vi "settings.vi"(8 "error in (no error)":errorcluster, 9 "low_resolution?":bool, 11 "reference in":refnum<class "Project Panels.lvclass">) -> (0 "error out":errorcluster, 3 "reference out":refnum<class "Project Panels.lvclass">)   [LabVIEW 2015, in "Project Panels.lvclass"]
uses:
  Project Panels.lvclass
  GUI Controller_llb/state.ctl
  GUI Controller_llb/GUI Controller.lvclass
  SYS/File Controller_llb/File Controller.lvclass
panel:
  out "Title":string
  in  "Number:":string
  in  "Service folder path:":path
  in  "TSR folder path:":path
  in  "not_tracking":bool caption="Notification"
  in  "not_items":bool caption="Notification"
  in  "Tab Control":T1(tab)
  in  "K5:":path
  in  "BB-PFT":path
  in  "RMR-ICU:":path
  in  "Pea Pod:":path
  in  "Bod Pod:":path
  in  "RMR:":path
  in  "CPET:":path
  in  "Fitmate:":path
  in  "K4b2:":path
  in  "K5:2":path caption="K5:"
  in  "BB-PFT 2":path caption="Body Box - PFT:"
  in  "RMR-ICU 2":path caption="RMR-ICU:"
  in  "Pea Pod: 2":path caption="Pea Pod:"
  in  "Bod Pod: 2":path caption="Bod Pod:"
  in  "RMR: 2":path caption="RMR:"
  in  "CPET: 2":path caption="CPET:"
  in  "Fitmate: 2":path caption="Fitmate:"
  in  "K4b2: 2":path caption="K4b2:"
  in  "PartsTracking:":path
  in  "Storage:":path
  in  "Products:":path
  out "StatusBar":string
  in  "Save Button":bool
  in  "Stop Button":bool
  # "Excel Files paths:"
  # "TSR settings:"
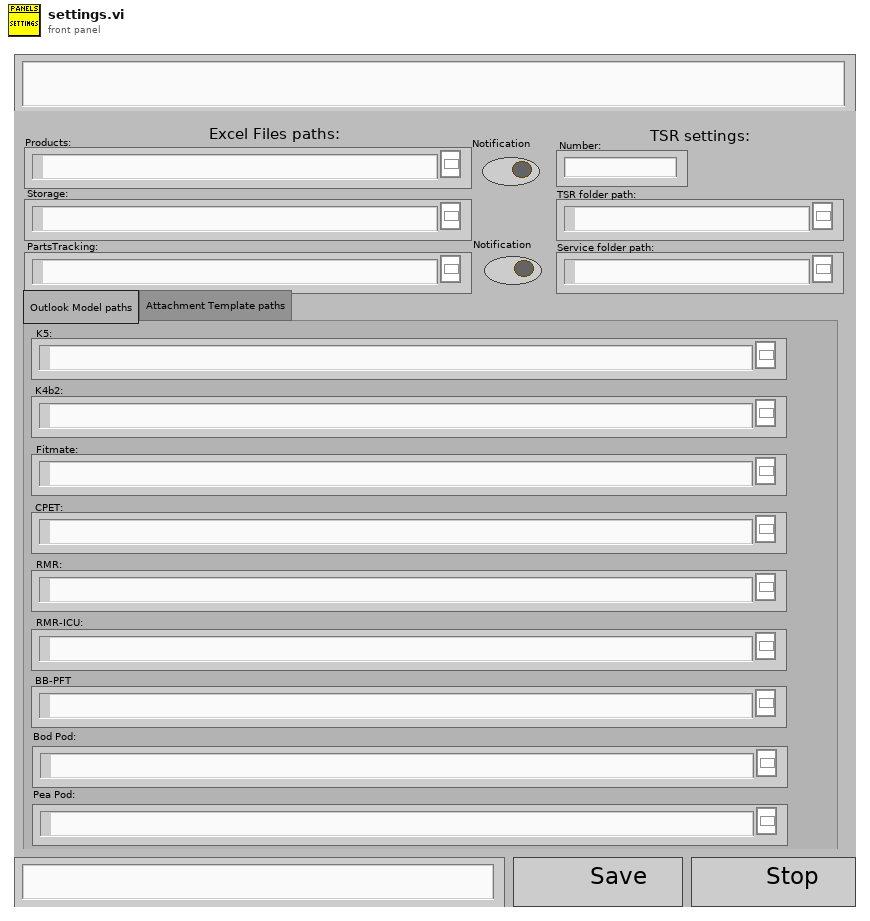
[diagram p1: front panel]
types:
  T1 = enum32{"Outlook Model paths", "Attachment Template paths"}
  T2 = typedef "GUI Controller.lvclass/state.ctl" = enum16{"initiate", "checkNotificationItems", "checkNotificationTracking", "operate", "updateFromFile", "stop"}
  T3 = enum16{"Always On", "Always Off", "Off While Running"}
  T4 = cluster{"number":string, "TSR_path":path, "service_path":path}
  T5 = typedef "Project Panels.lvclass/ObjectAttributesRef.ctl" = refnum<data-value>
  T6 = typedef "Project Panels.lvclass/ObjectAttributes.ctl" = cluster{"MyAttribute":dbl, "device_controller_ref":refnum<class "Devices Controller.lvclass">, "file_controller_ref":refnum<class "File Controller.lvclass">, "item_controller_ref":refnum<class "Items Controller.lvclass">, "item_tables":cluster{"checkIN":string[][], "checkOUT":string[][], "storage":string[][]}, "quickbook_table":cluster{"notes":string[][]}, "notification_controller_ref":refnum<class "Notification Controller.lvclass">, "partstracking_controller_ref":refnum<class "PartsTracking Controller.lvclass">, "product_tables":cluster{"k4b2":string[][], "fitmate":string[][], "RMR":string[][], "CPET":string[][], "BP":string[][], "PP":string[][], "k5":string[][], "bb-pft":string[][]}, "rowsColour":u32[], "low_resolution?":bool}
  T7 = cluster{"filePaths":path[], "outlookTemplatePaths":path[], "attachmentTemplatePaths":path[]}
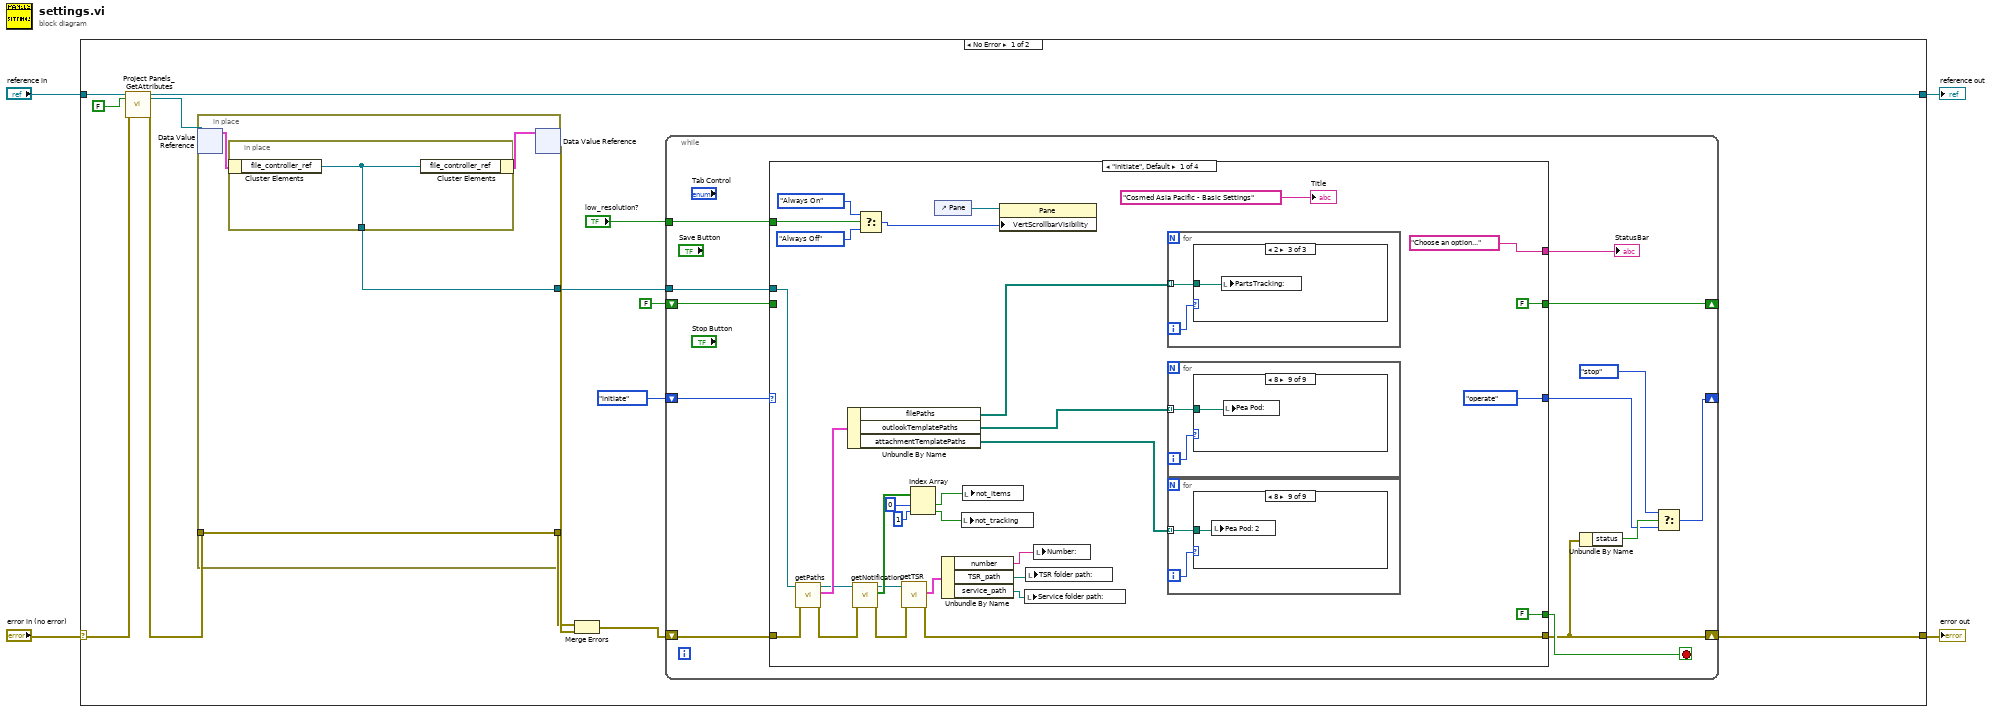
[diagram p0: block diagram]
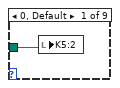
[diagram p2: hidden frame]
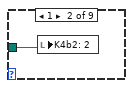
[diagram p3: hidden frame]
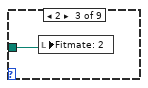
[diagram p4: hidden frame]
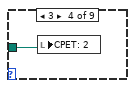
[diagram p5: hidden frame]
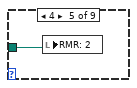
[diagram p6: hidden frame]
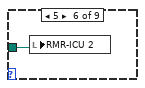
[diagram p7: hidden frame]
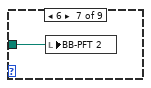
[diagram p8: hidden frame]
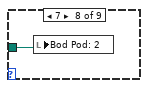
[diagram p9: hidden frame]
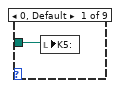
[diagram p10: hidden frame]
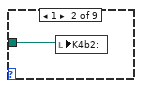
[diagram p11: hidden frame]
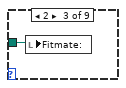
[diagram p12: hidden frame]
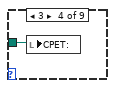
[diagram p13: hidden frame]
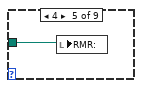
[diagram p14: hidden frame]
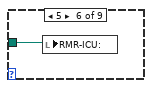
[diagram p15: hidden frame]
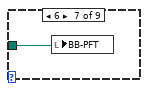
[diagram p16: hidden frame]
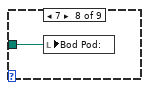
[diagram p17: hidden frame]
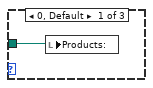
[diagram p18: hidden frame]
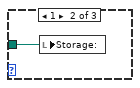
[diagram p19: hidden frame]
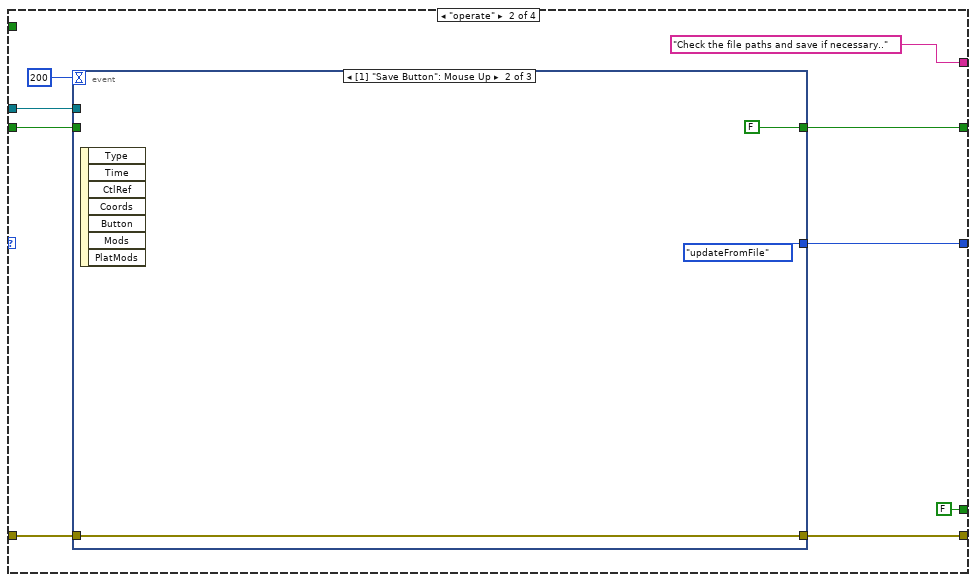
[diagram p20: hidden frame]
diagram:
  n1 = case shown="No Error" "error in (no error)" {
    selector: "error in (no error)" -> [w14 w191]
    tunnel: [w7 w191] -> w3
    tunnel: [w12 w190] -> w1
    tunnel: "reference in" -> [w16 w190]
    frame No Error {
      n2 = call "Project Panels_GetAttributes.vi"("reference in"=w16, "return data? (T)"=FALSE, "error in (no error)"=w14) -> ("reference out"=w12:refnum<class "Project Panels.lvclass">, "attributes ref"=w11:T5, "error out"=w13:errorcluster)  [unwired: 13 in, 1 out]
      n3 = in-place {
        in-place-border: w13 -> [w186]
        in-place-border: [w186] -> w17
        in-place-border: [w185] -> w8
        n4 = in-place-dvr #1(w11) -> (w187:T6)  [unwired: 1 out]
        n5 = in-place {
          in-place-border: [w189] -> w185
          n6 = in-place-cluster #2(w187) -> ("file_controller_ref"=w189:refnum<class "File Controller.lvclass">)
          n7 = in-place-cluster #2("file_controller_ref"=w189) -> (w188:T6)
        }
        n8 = in-place-dvr #1(w188) -> (w18:errorcluster)  [unwired: 1 out]
      }
      n9 = Merge Errors(w17, w18) -> (w10:errorcluster)
      n10 = while {
        shift-right: [w25] -> _
        shift-left: state."initiate" ("state") -> [w30]
        shift-right: [w27] -> w7
        shift-left: w10 -> [w31]
        tunnel: w8 -> [w24]
        shift-right: [w21] -> _
        shift-left: FALSE -> [w20]
        tunnel: "low_resolution?" -> [w19]
        stop <- w28 stop-if-true
        n11 = case shown="\"initiate\", Default" w30 {
          tunnel: w31 -> [w56 w95 w132 w159]
          tunnel: [w41 w94 w137 w158] -> w27
          tunnel: [state."operate" ("state") w91 state."operate" ("state") w157] -> w23
          tunnel: ["Choose an option..." ("Title") "Check the file paths and save if necessary.." ("Title") "Saving....." ("Title") "Stopped..." ("Title")] -> w29
          tunnel: [FALSE FALSE FALSE ("Save") w156] -> w28
          tunnel: w24 -> [w57 w92 w138 _]
          tunnel: [FALSE w90 TRUE FALSE] -> w21
          tunnel: w20 -> [_ w89 _ w160]
          tunnel: w19 -> [w35 _ _ _]
          frame "initiate", Default {
            n12 = call "getPaths.vi"("error in (no error)"=w56, "reference in"=w57) -> ("error out"=w49:errorcluster, "paths"=w55:T7, "reference out"=w50:refnum<class "File Controller.lvclass">)  [unwired: 7 in]
            n13 = Unbundle By Name(w55) -> ("filePaths"=w54:path[], "outlookTemplatePaths"=w53:path[], "attachmentTemplatePaths"=w52:path[])
            n14 = call "getNotification.vi"("error in (no error)"=w49, "reference in"=w50) -> ("error out"=w42:errorcluster, "not_setting"=w48:bool[], "reference out"=w43:refnum<class "File Controller.lvclass">)  [unwired: 7 in]
            n15 = Select(t=T3."Always On" ("Horizontal Scrollbar Visibility"), s=w35, f=T3."Always Off" ("Horizontal Scrollbar Visibility")) -> (s? t:f=w32:T3)
            n16 = call "getTSR.vi"("error in (no error)"=w42, "reference in"=w43) -> ("error out"=w41:errorcluster, "TSR"=w40:T4)  [unwired: 7 in, 1 out]
            n17 = Index Array(array=w48, index #1=0 ("index"), index #2=1 ("index")) -> (element #1=w45:bool, element #2=w44:bool)
            n18 = control-ref of="Pane"() -> (w36:refnum<vi>)
            n19 = Unbundle By Name(w40) -> ("number"=w39:string, "TSR_path"=w38:path, "service_path"=w37:path)
            n20 = local write "not_tracking"(w44) -> ()
            n21 = local write "not_items"(w45) -> ()
            n22 = property class="Pane"(reference=w36, "VertScrollbarVisibility"=w32) -> ()  [unwired: 1 in, 2 out]
            n23 = local write "Service folder path:"(w37) -> ()
            n24 = local write "TSR folder path:"(w38) -> ()
            n25 = local write "Number:"(w39) -> ()
            n26 = for {
              tunnel: w54 -> [w84] mode=indexing
              i -> [w85]
              n27 = case shown="2" w85 {
                tunnel: w84 -> [w86 w87 w88]
                frame 0, Default {
                  n28 = local write "Products:"(w86) -> ()
                }
                frame 1 {
                  n29 = local write "Storage:"(w87) -> ()
                }
                frame 2 {
                  n30 = local write "PartsTracking:"(w88) -> ()
                }
              }
            }
            n31 = for {
              tunnel: w53 -> [w73] mode=indexing
              i -> [w74]
              n32 = case shown="8" w74 {
                tunnel: w73 -> [w75 w76 w77 w78 w79 w80 w81 w82 w83]
                frame 0, Default {
                  n33 = local write "K5:"(w75) -> ()
                }
                frame 1 {
                  n34 = local write "K4b2:"(w76) -> ()
                }
                frame 2 {
                  n35 = local write "Fitmate:"(w77) -> ()
                }
                frame 3 {
                  n36 = local write "CPET:"(w78) -> ()
                }
                frame 4 {
                  n37 = local write "RMR:"(w79) -> ()
                }
                frame 5 {
                  n38 = local write "RMR-ICU:"(w80) -> ()
                }
                frame 6 {
                  n39 = local write "BB-PFT"(w81) -> ()
                }
                frame 7 {
                  n40 = local write "Bod Pod:"(w82) -> ()
                }
                frame 8 {
                  n41 = local write "Pea Pod:"(w83) -> ()
                }
              }
            }
            n42 = for {
              tunnel: w52 -> [w62] mode=indexing
              i -> [w63]
              n43 = case shown="8" w63 {
                tunnel: w62 -> [w64 w65 w66 w67 w68 w69 w70 w71 w72]
                frame 0, Default {
                  n44 = local write "K5:2"(w64) -> ()
                }
                frame 1 {
                  n45 = local write "K4b2: 2"(w65) -> ()
                }
                frame 2 {
                  n46 = local write "Fitmate: 2"(w66) -> ()
                }
                frame 3 {
                  n47 = local write "CPET: 2"(w67) -> ()
                }
                frame 4 {
                  n48 = local write "RMR: 2"(w68) -> ()
                }
                frame 5 {
                  n49 = local write "RMR-ICU 2"(w69) -> ()
                }
                frame 6 {
                  n50 = local write "BB-PFT 2"(w70) -> ()
                }
                frame 7 {
                  n51 = local write "Bod Pod: 2"(w71) -> ()
                }
                frame 8 {
                  n52 = local write "Pea Pod: 2"(w72) -> ()
                }
              }
            }
            "Title" <- "Cosmed Asia Pacific - Basic Settings" ("Title")
          }
          frame "operate" {
            n53 = event shown="[1] \"Save Button\": Mouse Up" {
              selector: _ -> [_ _ _]
              dyn-events: _ -> [_ _ _]
              timeout: 200 -> [_ _ _]
              tunnel: w95 -> [w99 w101 w104]
              tunnel: [w99 w101 w104] -> w94
              tunnel: w92 -> [_ _ _]
              tunnel: [state."operate" ("state") state."updateFromFile" ("state") state."stop" ("state")] -> w91
              tunnel: [w98 FALSE w105] -> w90
              tunnel: w89 -> [w98 _ w105]
              event Timeout {
                n54 = event-data() -> ()  [unwired: 1 in, 2 out]
              }
              event "Save Button": Mouse Up {
                n55 = event-data() -> ()  [unwired: 1 in, 7 out]
              }
              event "Stop Button": Mouse Up {
                n56 = event-data() -> ()  [unwired: 1 in, 7 out]
              }
            }
          }
          frame "updateFromFile" {
            n57 = flat-sequence {
              tunnel: w132 -> [w155]
              tunnel: [w155] -> w131
              frame #0 {
                n58 = local write "StatusBar"("Saving..." ("StatusBar")) -> ()
                n59 = Wait (ms)(milliseconds to wait=u32 1000) -> ()  [unwired: 1 out]
              }
            }
            n60 = Build Array("Products:", "Storage:", "PartsTracking:") -> (w139:path[])
            n61 = Build Array("K5:", "K4b2:", "Fitmate:", "CPET:", "RMR:", "RMR-ICU:", "BB-PFT", "Bod Pod:", "Pea Pod:") -> (w140:path[])
            n62 = Build Array("K5:2", "K4b2: 2", "Fitmate: 2", "CPET: 2", "RMR: 2", "RMR-ICU 2", "BB-PFT 2", "Bod Pod: 2", "Pea Pod: 2") -> (w141:path[])
            n63 = call "setPaths.vi"("reference in"=w138, "filePaths"=w139, "outlookTemplatePaths"=w140, "attachmentTemplatePaths"=w141, "error in (no error)"=w131) -> ("reference out"=w127:refnum<class "File Controller.lvclass">, "error out"=w126:errorcluster)  [unwired: 9 in]
            n64 = Build Array("not_items", "not_tracking") -> (w128:bool[])
            n65 = Bundle By Name(cluster=T4 {"number"="", "TSR_path"=path "", "service_path"=path ""} ("TSR"), "number"="Number:", "TSR_path"="TSR folder path:", "service_path"="Service folder path:") -> (w107:T4)
            n66 = call "setNotificationSettings.vi"("error in (no error)"=w126, "not_settings"=w128, "reference in"=w127) -> ("error out"=w115:errorcluster, "reference out"=w113:refnum<class "File Controller.lvclass">)  [unwired: 7 in]
            n67 = call "setTSR.vi"("error in (no error)"=w115, "TSR"=w107, "reference in"=w113) -> ("error out"=w114:errorcluster, "reference out"=w112:refnum<class "File Controller.lvclass">)  [unwired: 7 in]
            n68 = call "saveData.vi"("error in (no error)"=w114, "reference in"=w112) -> ("error out"=w137:errorcluster)  [unwired: 8 in, 1 out]
          }
          frame "stop" {
            n69 = Unbundle By Name(w159) -> ("status"=w162:bool)
            n70 = case shown="False" w162 {
              tunnel: w159 -> [w170 w181]
              tunnel: w160 -> [w171 _]
              tunnel: [w169 w181] -> w158
              tunnel: [w166 state."initiate" ("state")] -> w157
              tunnel: [w164 TRUE ("Save")] -> w156
              frame False {
                n71 = case shown="False" w171 {
                  tunnel: w170 -> [w176 w177]
                  tunnel: [w176 w177] -> w169
                  tunnel: [w174 FALSE ("Save")] -> w165
                  frame False {
                    n72 = Two Button Dialog(message="The panel will be closed without saving the data. Do you want to save the data?", 1:"Not Save" ("F button name (\"Cancel\")"), 2:"Save" ("T button name (\"OK\")")) -> (T button?=w174:bool)
                  }
                  frame True {
                  }
                }
                n73 = Not(x=w165) -> (.not. x?=w164:bool)
                n74 = Select(t=state."updateFromFile" ("state"), s=w165, f=state."stop" ("state")) -> (s? t:f=w166:T2)
              }
              frame True {
                n75 = Unbundle By Name(w181) -> ("source"=w182:string)
                n76 = Concatenate Strings("An Error occur: " ("message"), w182) -> (w184:string)
                n77 = One Button Dialog(message=w184) -> ()  [unwired: 1 in, 1 out]
              }
            }
          }
        }
        "StatusBar" <- w29
        n78 = Unbundle By Name(w27) -> ("status"=w26:bool)
        n79 = Select(t=state."stop", s=w26, f=w23) -> (s? t:f=w25:T2)
      }
    }
    frame Error {
    }
  }
  "error out" <- w3
  "reference out" <- w1
